vi "Display Units.vi"(8 "error in (no error)":errorcluster, 11 "VISA resource name":refnum<visa-resource-name>) -> (0 "error out":errorcluster, 2 "Units":string, 3 "VISA resource name out":refnum<visa-resource-name>)   [LabVIEW 2009, in "Newport 1830-C.lvlib"]
doc: "Reads units from instrument and ouputs symbol as a string."
uses:
  Newport 1830-C.lvlib
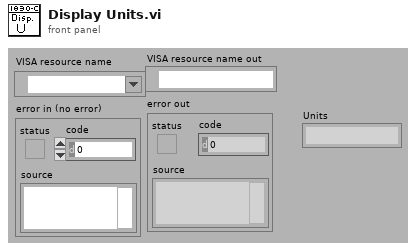
[diagram p1: front panel]
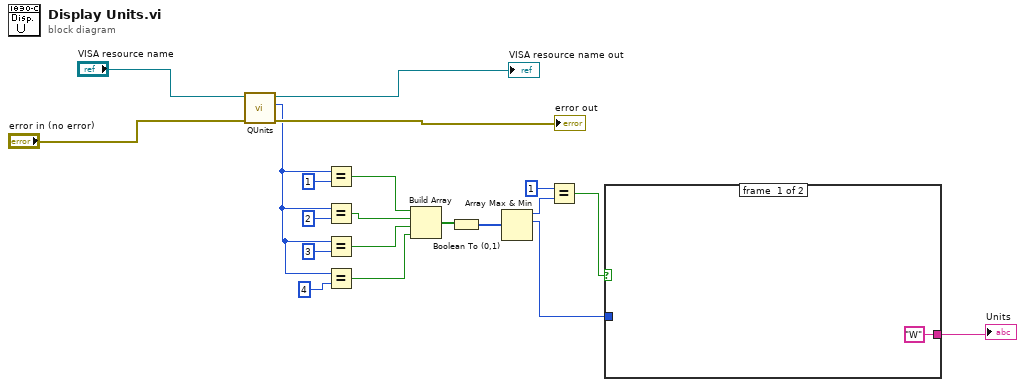
[diagram p0: block diagram]
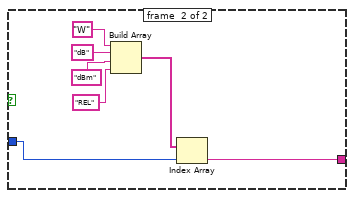
[diagram p2: hidden frame]
diagram:
  n1 = call "QUnits.vi"("error in (no error)"="error in (no error)", "VISA resource name"="VISA resource name") -> ("error out"=→"error out":errorcluster, "output"=w16:i32, "VISA resource name out"=→"VISA resource name out":refnum<visa-resource-name>)  [unwired: 7 in]
  n2 = Equal?(x=w16, y=1) -> (x = y?=w11:bool)
  n3 = Equal?(x=w16, y=2) -> (x = y?=w10:bool)
  n4 = Equal?(x=w16, y=3) -> (x = y?=w9:bool)
  n5 = Equal?(x=w16, y=4) -> (x = y?=w8:bool)
  n6 = Build Array(w11, w10, w9, w8) -> (w7:bool[])
  n7 = Boolean To (0,1)(Boolean=w7) -> (0, 1=w6:i16[])
  n8 = Array Max & Min(array=w6) -> (max value=w3:i16, max index (indices)=w5:i32)  [unwired: 2 out]
  n9 = Equal?(x=i16 1, y=w3) -> (x = y?=w1:bool)
  n10 = case shown="True" w1 {
    tunnel: w5 -> [_ w23]
    tunnel: ["W" w22] -> w4
    frame #0 {
    }
    frame #1 {
      n11 = Build Array("W", "dB", "dBm", "REL") -> (w24:string[])
      n12 = Index Array(array=w24, index=w23) -> (element=w22:string)
    }
  }
  "Units" <- w4
